vi "Set Alignment.vi"(0 "shared in":refnum<class "niUSRP Rx Core v1 FPGA.lvclass">=refnum, 5 "align":refnum<class "niVST Shared Alignment v1 FPGA.lvclass">=refnum) -> (4 "shared out":refnum<class "niUSRP Rx Core v1 FPGA.lvclass">)   [LabVIEW 2023]
uses:
  <instrlib>/niUSRP/Reference FPGA/Rx Core/niUSRP Rx Core v1 FPGA.lvclass
  <instrlib>/niVST/Reference FPGA/FPGA/Shared/v1/Alignment/niVST Shared Alignment v1 FPGA.lvclass
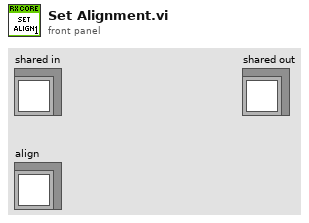
[diagram p1: front panel]
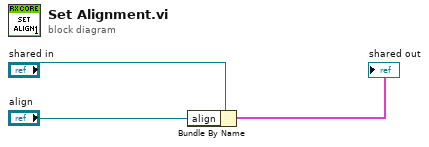
[diagram p0: block diagram]
diagram:
  n1 = Bundle By Name(cluster="shared in", "align"="align") -> (→"shared out":cluster{})
